vi "SetCurrentControl.vi"(0 "handle in":i32, 1 "UnitAddress(0)":u16, 2 "MotNr(0)":u8, 5 "error in(no error)":errorcluster, 7 "I Control":T1={"PowerDownDelay (500)"=500, "PowerDown (0%)"=enum."0%", "Standing (50%)"=enum."50%", "Running (75%)"=enum."75%", "Accelerating (100%)"=enum."100%"}) -> (14 "handle out":i32, 19 "error out":errorcluster)   [LabVIEW 2014, in "Sixpack - Driver.lvlib"]
doc: "ACHTUNG: PowerDownDelay wird auch für das Testnull-Delay (Befehl SetMotorParameters, Flag MT_DELAYTESTNULL) benötigt!\n\nBietet die Möglichkeit den Motorstrom in Abhängigkeit der ausgeführten Aktion zu setzen. Hierbei können, in einer prozentualen Abstufung von 100%, 75%, 50%, 38%, 25%, 19%, 13%, 9% und 0%, die jeweiligen Stromwerte für die unten genannten Zustände gesetzt werden.\n\nHinweis zur Energieeinsparung: \nEine deutliche Reduktion der gesamten Stromaufnahme kann erreicht werden, indem PowerDownCurrent für alle (ungenutzten) Motorausgänge auf 0%gesetzt wird.\n\nCMD $11\nP0 MotorNr (0...5)\nPowerDownCurrent: Power Down- Strom.\nStandingCurrent: Strom bei stehendem Motor (vor Ablauf von PowerDownDelay).\nRunningCurrent: Strom während konstanter Geschwindigkeit\nAccelerationCurrent: Strom während Beschleunigung\nPowerDownDelay: (1..65535) Power Down- Verzögerungszeit. \nEinstellung in Schritten zu 2 ms (Wartezeit = PowerDownDelay * 2 ms)."
uses:
  Sixpack - Driver.lvlib
  Current Control.ctl
  Current.ctl
  DLL/PackDLL.dll
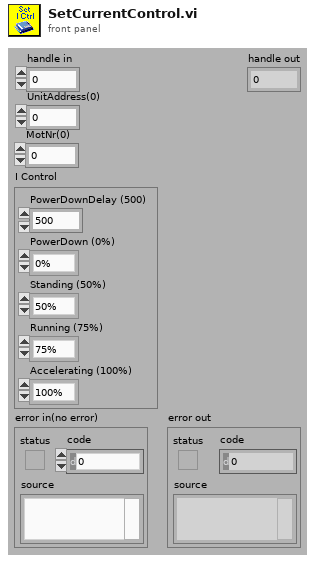
[diagram p1: front panel]
types:
  T1 = typedef "Sixpack - Driver.lvlib/Current Control.ctl" = cluster{"PowerDownDelay (500)":u16, "PowerDown (0%)":T2, "Standing (50%)":T2, "Running (75%)":T2, "Accelerating (100%)":T2}
  T2 = typedef "Sixpack - Driver.lvlib/Current.ctl" = enum8{"100%", "75%", "50%", "38%", "25%", "19%", "13%", "9%", "0%"}
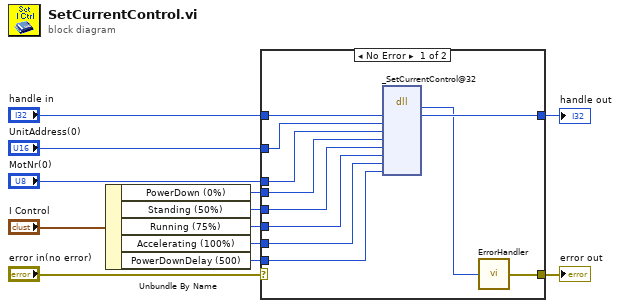
[diagram p0: block diagram]
diagram:
  n1 = Unbundle By Name("I Control") -> ("PowerDown (0%)"=w5:T2, "Standing (50%)"=w4:T2, "Running (75%)"=w3:T2, "Accelerating (100%)"=w2:T2, "PowerDownDelay (500)"=w1:u16)
  n2 = case shown="No Error" "error in(no error)" {
    selector: "error in(no error)" -> [_ w24]
    tunnel: "handle in" -> [w23 w25]
    tunnel: [w22 w25] -> w11
    tunnel: "UnitAddress(0)" -> [w21 _]
    tunnel: "MotNr(0)" -> [w20 _]
    tunnel: w4 -> [w19 _]
    tunnel: w3 -> [w18 _]
    tunnel: w2 -> [w17 _]
    tunnel: w1 -> [w16 _]
    tunnel: w5 -> [w15 _]
    tunnel: [w13 w24] -> w8
    frame No Error {
      n3 = dll-call lib="D:/CS-Source/LV2014/GPL/instr.lib/SixPack/PackDLL/DLL/PackDLL.dll" fn="_SetCurrentControl@32" label="SetPeakCurrent"("HANDLE"=w23, "UnitAddress"=w21, "MotNr"=w20, "PowerDownCurrent"=w15, "StandingCurrent"=w19, "RunningCurrent"=w18, "AcceleratingCurrent"=w17, "PowerDownDelay"=w16) -> ("BOOLEAN"=w14:i8, "HANDLE"=w22:i32)  [unwired: 10 in, 2 out]
      n4 = call "ErrorHandler.vi"("BOOLEAN"=w14) -> ("error out"=w13:errorcluster)
    }
    frame Error {
    }
  }
  "handle out" <- w11
  "error out" <- w8
